vi "Mcad15 Variable Names.vi"(0 "Eval Regions":string[](array[string])) -> (7 "Name":string[](array[string]), 8 "Name.Sub":string[](array[string]))   [LabVIEW 2012, in "Design Server.lvlib"]
uses:
  Design Server.lvlib
panel:
  in  "regular expression":string="<ml:id xml:space=\"preserve\" subscript=\"[~\"<>]*\""
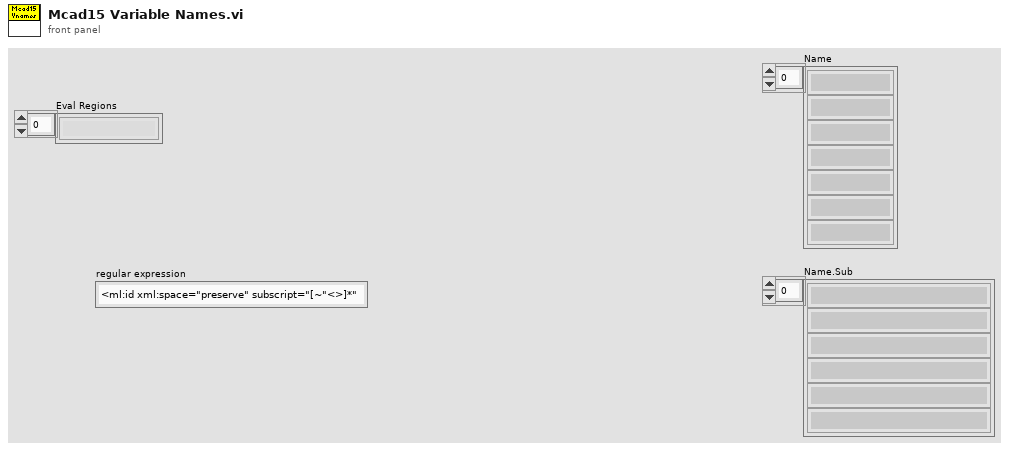
[diagram p1: front panel]
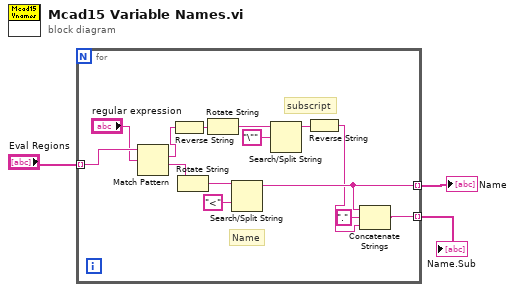
[diagram p0: block diagram]
diagram:
  n1 = for {
    tunnel: [w6] -> w2 mode=indexing
    tunnel: "Eval Regions" -> [w17] mode=indexing
    tunnel: [w4] -> w1 mode=indexing
    # "Name"
    # "subscript"
    n2 = Match Pattern(string=w17, regular expression="regular expression") -> (match substring=w10:string, after substring=w8:string)  [unwired: 1 in, 2 out]
    n3 = Reverse String(1:w10) -> (0:w14:string)
    n4 = Rotate String(1:w8) -> (0:w12:string)
    n5 = Rotate String(1:w14) -> (0:w13:string)
    n6 = Search/Split String(string=w12, search string/char (-)="<") -> (substring before match=w6:string)  [unwired: 1 in, 2 out]
    n7 = Search/Split String(string=w13, search string/char (-)="\"") -> (substring before match=w15:string)  [unwired: 1 in, 2 out]
    n8 = Reverse String(1:w15) -> (0:w5:string)
    n9 = Concatenate Strings(w6, "." ("string"), w5) -> (w4:string)
  }
  "Name" <- w2
  "Name.Sub" <- w1
